vi "Read a_hDevice.vi"(8 "error in (no error)":errorcluster, 11 "Avantes in":refnum<class "Avantes.lvclass">) -> (0 "error out":errorcluster, 2 "a_hDevice":i32, 3 "Avantes out":refnum<class "Avantes.lvclass">)   [LabVIEW 2020, in "Avantes.lvclass"]
uses:
  <instrlib>/Classes/CCD/Avantes/Avantes.lvclass
  <instrlib>/Classes/CCD/Avantes/Avantes.lvclass/Avantes.ctl
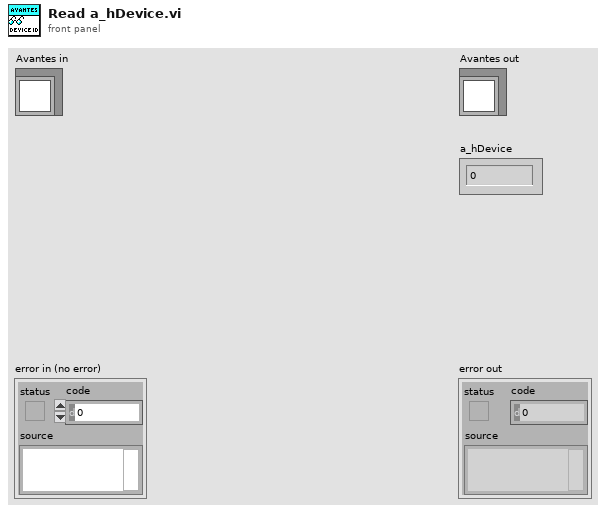
[diagram p1: front panel]
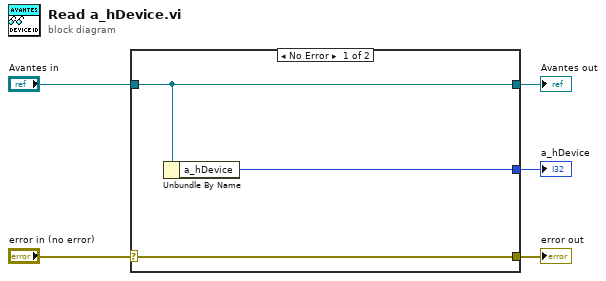
[diagram p0: block diagram]
diagram:
  n1 = case shown="No Error" "error in (no error)" {
    selector: "error in (no error)" -> [w8 w9]
    tunnel: [w8 w9] -> w4
    tunnel: [w7 w10] -> w2
    tunnel: "Avantes in" -> [w7 w10]
    tunnel: [w6 _] -> w1
    frame No Error {
      n2 = Unbundle By Name(w7) -> ("a_hDevice"=w6:i32)
    }
    frame Error {
    }
  }
  "error out" <- w4
  "Avantes out" <- w2
  "a_hDevice" <- w1
